vi "未命名3.vi"() -> ()   [LabVIEW 2020]
panel:
  in  "路径":path
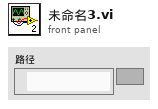
[diagram p1: front panel]
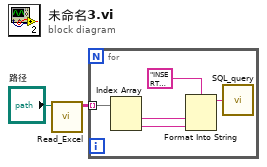
[diagram p0: block diagram]
diagram:
  n1 = call "Read_Excel.vi"("路径"="路径") -> ("表格控件"=w1:string[][])  [unwired: 10 in]
  n2 = for {
    tunnel: w1 -> [w5] mode=indexing
    n3 = Index Array(array=w5) -> (element #1=w4:string, element #2=w3:string)  [unwired: 2 in]
    n4 = Format Into String(format string="INSERT INTO [SanliServer].[dbo].[不合格代码] ([不合格代码], [不合格原因]) OUTPUT INSERTED.[不合格代码], INSERTED.[不合格原因] VALUES (N'%s', N'%s')" ("SQL query"), w4, w3) -> (resulting string=w6:string)  [unwired: 2 in, 1 out]
    n5 = call "SQL_query.vi"("SQL query"=w6) -> ()  [unwired: 3 in, 2 out]
  }
